vi "Activate.vi"(1 "Button":T1(ring)) -> (0 "BooleanAddress":u16)   [LabVIEW 2010, in "FTC.lvlib" / "Remote Interface.lvlib"]
uses:
  Remote Interface.lvlib
  CLIB/CRef/CRef.lvlib
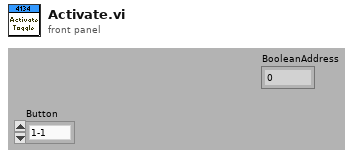
[diagram p1: front panel]
types:
  T1 = enum16{"1-1", "1-2", "1-3", "1-4", "1-5", "1-6", "1-7", "1-8", "1-9", "1-10", "1-11", "1-12", "2-1", "2-2", "2-3", "2-4", "2-5", "2-6", "2-7", "2-8", "2-9", "2-10", "2-11", "2-12", "NXT-L", "NXT-R", "NXT-E", "1-U", "1-UR", "1-R", "1-DR", "1-D", "1-DL", "1-L", "1-UL", "2-U", "2-UR", "2-R", "2-DR", "2-D", "2-DL", "2-L", "2-UL"}
  T2 = typedef "CRef.lvlib/I32 CReference.ctl" = cluster{"Generic CRef Address":u16, "Type":enum8{"Null", "Boolean", "U8", "I8", "U16", "I16", "U32", "I32", "U64", "I64", "Single", "Double", "Extended", "CSG", "CDB", "CXT", "Invalid Def", "U8(Def)", "I8(Def)", "U16(Def)", "I16(Def)", "U32(Def)", "I32(Def)"}}
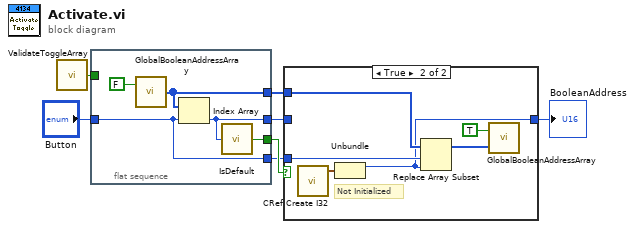
[diagram p0: block diagram]
diagram:
  n1 = call "ValidateToggleArray.vi"() -> ("Valid?"=w7:bool)
  n2 = flat-sequence {
    tunnel: w7 -> [_]
    tunnel: "Button" -> [w10]
    tunnel: [w11] -> w6
    tunnel: [w10] -> w5
    tunnel: [w9] -> w4
    tunnel: [w8] -> w3
    frame #0 {
      n3 = call "GlobalBooleanAddressArray.vi"("Write?"=FALSE) -> ("Array"=w9:u16[])  [unwired: 1 in]
      n4 = Index Array(array=w9, index=w10) -> (element=w8:u16)
      n5 = call "IsDefault.vi"("Address"=w8) -> ("Default?"=w11:bool)
    }
  }
  n6 = case shown="True" w6 {
    tunnel: w5 -> [_ w18]
    tunnel: w4 -> [_ w17]
    tunnel: [w13 w14] -> w2
    tunnel: w3 -> [w13 _]
    frame False {
      # "Initialized"
    }
    frame True {
      # "Not Initialized"
      n7 = call "CRef Create I32.vi"() -> ("I32 CReference"=w15:T2)  [unwired: 5 in]
      n8 = Unbundle(w15) -> ("Generic CRef Address"=w14:u16)  [unwired: 1 out]
      n9 = Replace Array Subset(array=w17, new element=w14, index=w18) -> (w16:u16[])
      n10 = call "GlobalBooleanAddressArray.vi"("Write Array"=w16, "Write?"=TRUE) -> ()  [unwired: 1 out]
    }
  }
  "BooleanAddress" <- w2
